vi "BrakingState.vi"(8 "error in (no error)":errorcluster, 9 "Cluster in":T2, 10 "Enum in":T1, 11 "Double":dbl) -> (0 "error out":errorcluster, 2 "Cluster":T2, 3 "Enum":T1)   [LabVIEW 2018]
uses:
  Type_Def/Type_Def Actuator Controls.ctl
  Type_Def/Type_Def ControlState.ctl
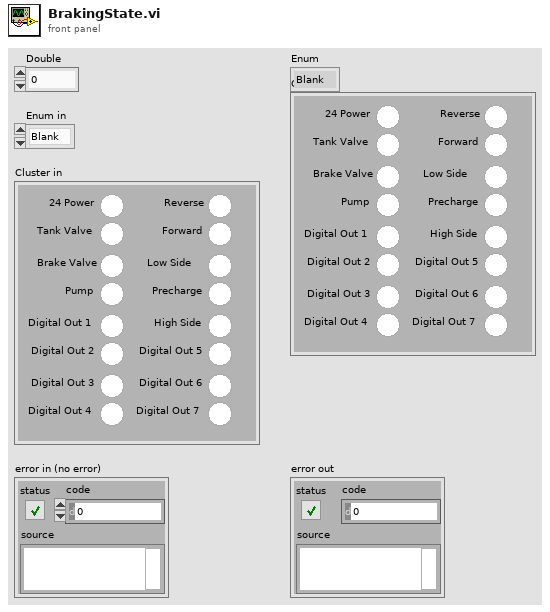
[diagram p1: front panel]
types:
  T1 = typedef "Type_Def ControlState.ctl" = enum16{"Blank", "Systems Check", "Idle", "Ready", "Pushing", "CrawlingPrecharge", "Braking", "Fault", "Boot Up", "Unpowered", "Crawling", "Shutdown", "Service Push", "Service Wait", "Vent", "Precharge", "Cooldown"}
  T2 = typedef "Type_Def Actuator Controls.ctl" = cluster{"Reverse ":bool, "Forward":bool, "Low Side":bool, "Precharge":bool, "High Side":bool, "Digital Out 5":bool, "Digital Out 6":bool, "Digital Out 7 ":bool, "24 Power":bool, "Tank Valve ":bool, "Brake Valve":bool, "Pump":bool, "Digital Out 1 ":bool, "Digital Out 2":bool, "Digital Out 3":bool, "Digital Out 4 ":bool}
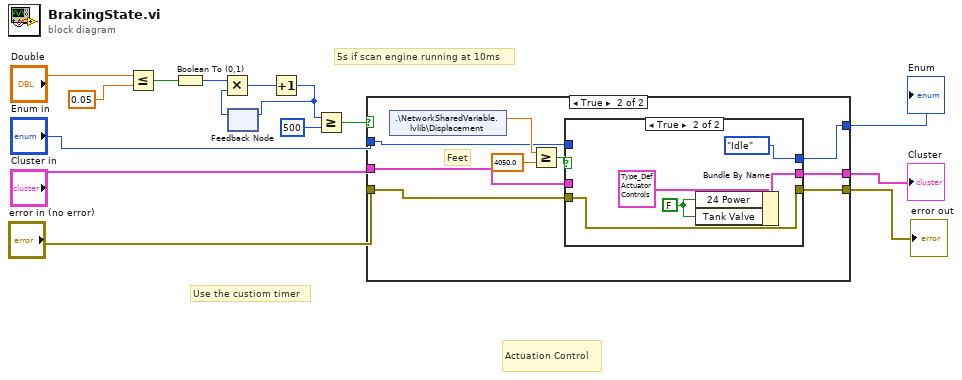
[diagram p0: block diagram]
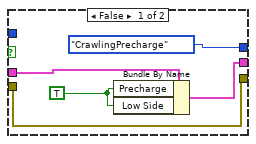
[diagram p3: hidden frame]
diagram:
  # "5s if scan engine running at 10ms"
  # "Use the custiom timer"
  # "Actuation Control"
  n1 = Less Or Equal?(x="Double", y=0.05) -> (x <= y?=w9:bool)
  n2 = Boolean To (0,1)(Boolean=w9) -> (0, 1=w10:i16)
  n3 = feedback #1() -> (w15:i16)  [unwired: 1 in]
  n4 = Multiply(x=w10, y=w15) -> (x*y=w11:i16)
  n5 = Increment(x=w11) -> (x+1=w14:i16)
  n6 = feedback-in #1(w14) -> ()
  n7 = Greater Or Equal?(x=w14, y=i16 500) -> (x >= y?=w12:bool)
  n8 = case shown="True" w12 {
    tunnel: "Enum in" -> [w18 w19]
    tunnel: [w18 w20] -> w2
    tunnel: "Cluster in" -> [w17 w21]
    tunnel: [w17 w22] -> w4
    tunnel: [w16 w24] -> w5
    tunnel: "error in (no error)" -> [w16 w23]
    frame False {
      # "Pass the value for the next state through"
    }
    frame True {
      # "Feet"
      n9 = shared-variable ".\\NetworkSharedVariable.lvlib\\Displacement"() -> (w27:dbl)  [unwired: 1 in, 1 out]
      n10 = Greater Or Equal?(x=w27, y=4050.0) -> (x >= y?=w25:bool)
      n11 = case shown="True" w25 {
        tunnel: [w31 w34] -> w24
        tunnel: w23 -> [w31 w34]
        tunnel: [w29 w35] -> w22
        tunnel: w21 -> [w30 _]
        tunnel: [Type_Def_ControlState."CrawlingPrecharge" Type_Def_ControlState."Idle"] -> w20
        tunnel: w19 -> [_ _]
        frame False {
          w28 = TRUE ("Digital Out 5")
          n12 = Bundle By Name(cluster=w30, "Precharge"=w28, "Low Side"=w28) -> (w29:T2)
        }
        frame True {
          w33 = FALSE ("Digital Out 5")
          n13 = Bundle By Name(cluster=T2 {"Reverse "=TRUE, "Forward"=TRUE, "Low Side"=TRUE, "Precharge"=TRUE, "High Side"=TRUE, "Digital Out 5"=TRUE, "Digital Out 6"=TRUE, "Digital Out 7 "=TRUE, "24 Power"=TRUE, "Tank Valve "=TRUE, "Brake Valve"=TRUE, "Pump"=TRUE, "Digital Out 1 "=TRUE, "Digital Out 2"=TRUE, "Digital Out 3"=TRUE, "Digital Out 4 "=TRUE}, "24 Power"=w33, "Tank Valve"=w33) -> (w35:T2)
        }
      }
    }
  }
  "error out" <- w5
  "Cluster" <- w4
  "Enum" <- w2
